vi "Display.vi"(8 "error in (no error)":errorcluster, 11 "DriverMaster in":refnum<class "DriverMaster.lvclass">) -> (0 "error out":errorcluster, 3 "DriverMaster out":refnum<class "DriverMaster.lvclass">)   [LabVIEW 2014, in "DriverMaster.lvlib" / "DriverMaster.lvclass"]
uses:
  DriverMaster.lvclass
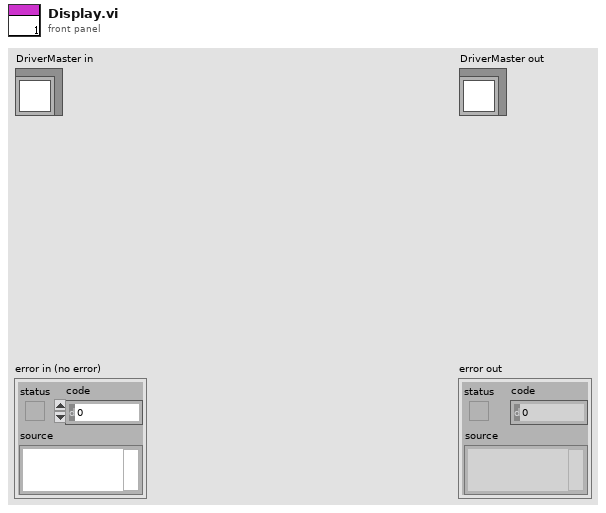
[diagram p1: front panel]
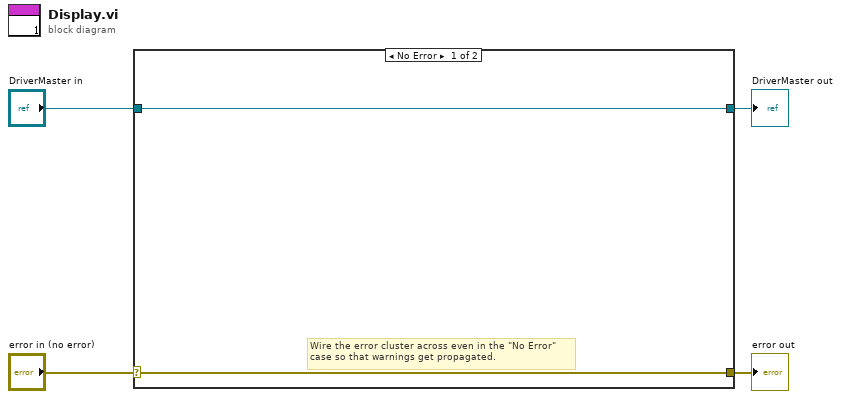
[diagram p0: block diagram]
diagram:
  n1 = case shown="No Error" "error in (no error)" {
    selector: "error in (no error)" -> [w5 w8]
    tunnel: [w5 w8] -> w3
    tunnel: [w6 w7] -> w1
    tunnel: "DriverMaster in" -> [w6 w7]
    frame No Error {
      # "Wire the error cluster across even in the \"No Error\"\ncase so that warnings get propagated."
    }
    frame Error {
    }
  }
  "error out" <- w3
  "DriverMaster out" <- w1
